vi "Set Security Level CORE.vi"(8 "error in (no error)":errorcluster, 9 "Set or Clear":T1, 10 "Security Level":T2, 11 "Door Alarm in":refnum<class "Door Alarm.lvclass">) -> (0 "error out":errorcluster, 2 "Last Action Performed":string, 3 "Door Alarm out":refnum<class "Door Alarm.lvclass">)   [LabVIEW 2020, in "Door Alarm.lvclass"]
uses:
  Door Alarm.lvclass
  Security System/Security Level.ctl
  Security System/Set or Clear.ctl
  Door Alarm.lvclass/Door Alarm.ctl
  Security System/Security System.lvclass
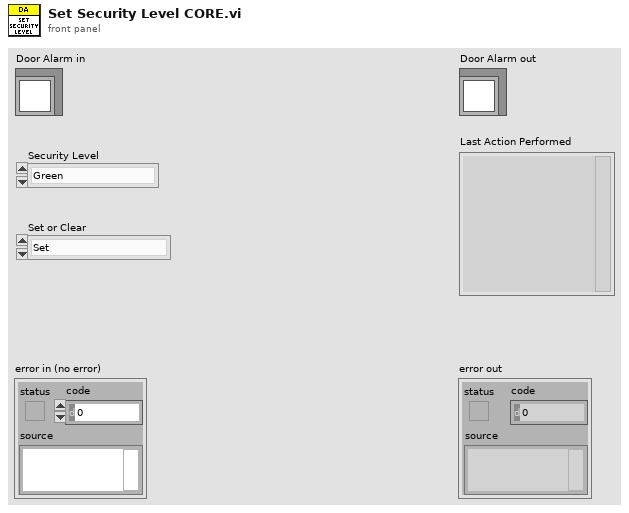
[diagram p1: front panel]
types:
  T1 = typedef "Security System.lvclass/Set or Clear.ctl" = enum16{"Set", "Clear"}
  T2 = typedef "Security System.lvclass/Security Level.ctl" = enum16{"Green", "Yellow", "Orange", "Red"}
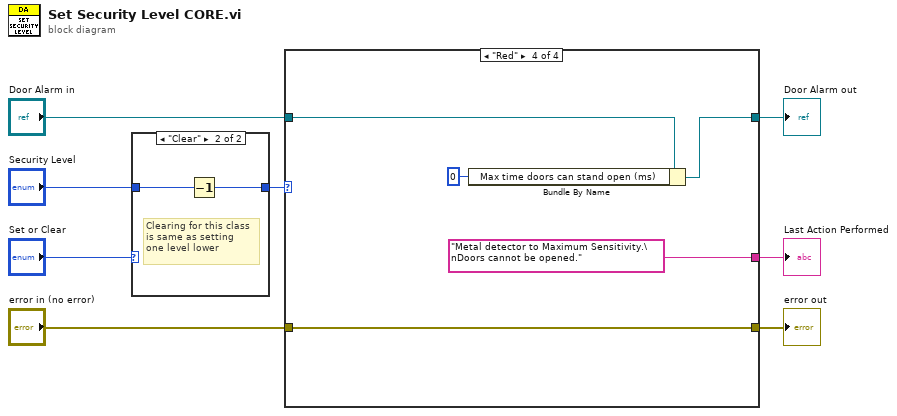
[diagram p0: block diagram]
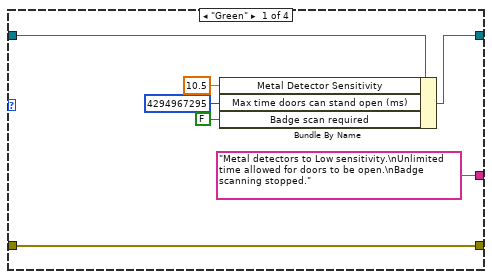
[diagram p2: hidden frame]
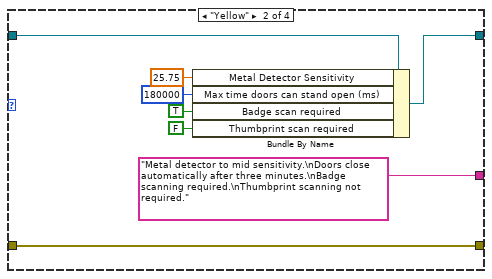
[diagram p3: hidden frame]
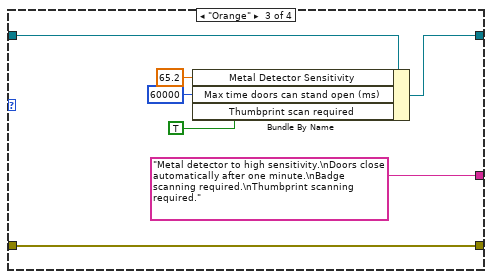
[diagram p4: hidden frame]
diagram:
  n1 = case shown="\"Clear\"" "Set or Clear" {
    tunnel: "Security Level" -> [w9 w11]
    tunnel: [w9 w10] -> w6
    frame "Set" {
    }
    frame "Clear" {
      # "Clearing for this class\nis same as setting\none level lower"
      n2 = Decrement(x=w11) -> (x-1=w10:T2)
    }
  }
  n3 = case shown="\"Red\"" w6 {
    tunnel: "Door Alarm in" -> [w18 w26 w33 w38]
    tunnel: "error in (no error)" -> [w12 w20 w28 w35]
    tunnel: [w17 w25 w32 w37] -> w3
    tunnel: ["Metal detectors to Low sensitivity.\nUnlimited time allowed for doors to be open.\nBadge scanning stopped." "Metal detector to mid sensitivity.\nDoors close automatically after three minutes.\nBadge scanning required.\nThumbprint scanning not required." "Metal detector to high sensitivity.\nDoors close automatically after one minute.\nBadge scanning required.\nThumbprint scanning required." "Metal detector to Maximum Sensitivity.\nDoors cannot be opened."] -> w2
    tunnel: [w12 w20 w28 w35] -> w1
    frame "Green" {
      n4 = Bundle By Name(cluster=w18, "Metal Detector Sensitivity"=10.5, "Max time doors can stand open (ms)"=u32 4294967295, "Badge scan required"=FALSE) -> (w17:refnum<class "Door Alarm.lvclass">)
    }
    frame "Yellow" {
      n5 = Bundle By Name(cluster=w26, "Metal Detector Sensitivity"=25.75, "Max time doors can stand open (ms)"=u32 180000, "Badge scan required"=TRUE, "Thumbprint scan required"=FALSE) -> (w25:refnum<class "Door Alarm.lvclass">)
    }
    frame "Orange" {
      n6 = Bundle By Name(cluster=w33, "Metal Detector Sensitivity"=65.2, "Max time doors can stand open (ms)"=u32 60000, "Thumbprint scan required"=TRUE) -> (w32:refnum<class "Door Alarm.lvclass">)
    }
    frame "Red" {
      n7 = Bundle By Name(cluster=w38, "Max time doors can stand open (ms)"=u32 0) -> (w37:refnum<class "Door Alarm.lvclass">)
    }
  }
  "error out" <- w1
  "Door Alarm out" <- w3
  "Last Action Performed" <- w2
